vi "Build Report String.vi"(8 "error in (no error)":errorcluster, 10 "Report Data":T1, 11 "Control Assertion in":refnum<class "Control Assertion.lvclass">) -> (0 "error out":errorcluster, 2 "Report String":string, 3 "Control Assertion out":refnum<class "Control Assertion.lvclass">)   [LabVIEW 2020, in "MacroAssert.lvlib" / "Control Assertion.lvclass"]
doc: "Builds a string using <B>Step</B> and <B>Report Data</B> to be included in a report."
uses:
  Control Assertion.lvclass
  Control Assertion.lvclass/Control Assertion.ctl
  CTLs/Report Data.ctl
  MacroAssert.lvlib
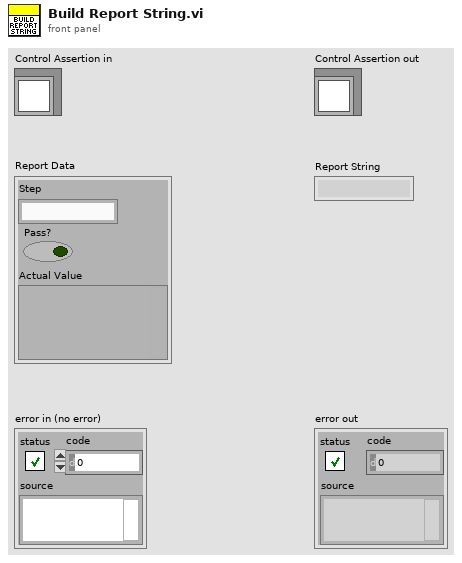
[diagram p1: front panel]
types:
  T1 = typedef "MacroAssert.lvlib/Report Data.ctl" = cluster{"Step":string, "Pass?":bool, "Actual Value":variant}
  T2 = typedef "MacroAssert.lvlib/Step Type V3.ctl" = enum16{"Mouse Move", "Mouse Click", "Key Press", "Wait", "Mouse Down", "Mouse Up", "Key Down", "Key Up", "Test Assertion", "Maximize Window", "Restore Window", "Minimize Window", "Close Window", "Bring Window to Front", "Send Window to Back"}
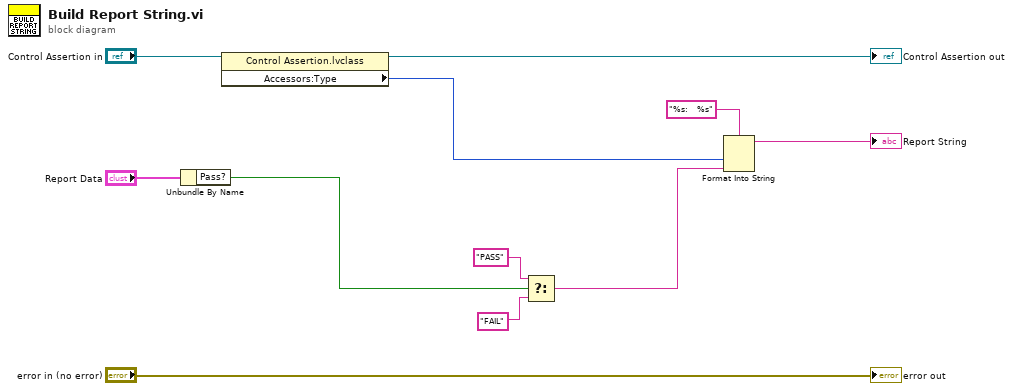
[diagram p0: block diagram]
diagram:
  n1 = Unbundle By Name("Report Data") -> ("Pass?"=w3:bool)
  n2 = property class="Control Assertion.lvclass"(reference="Control Assertion in") -> (reference out=→"Control Assertion out":refnum<class "Control Assertion.lvclass">, "Accessors:Type"=w1:T2)  [unwired: 1 in, 1 out]
  n3 = Select(t="PASS", s=w3, f="FAIL") -> (s? t:f=w8:string)
  n4 = Format Into String(format string="%s:   %s", w1, w8) -> (resulting string=→"Report String":string)  [unwired: 2 in, 1 out]
  "error out" <- "error in (no error)"
